vi "onSubscribe.vi"(6 "timeout (100ms)":i32=100, 8 "error in (no error)":errorcluster, 10 "SUBSCRIBE":refnum<class "SUBSCRIBE.lvclass">, 11 "MQTT_Base in":refnum<class "MQTT_Base.lvclass">) -> (0 "error out":errorcluster, 2 "SUBACK":refnum<class "SUBACK.lvclass">, 3 "MQTT_Base out":refnum<class "MQTT_Base.lvclass">)   [LabVIEW 2013, in "MQTT Base.lvlib" / "MQTT_Base.lvclass"]
uses:
  MQTT_Base.lvclass
  <vilib>/LabVIEW Open Source Project/MQTT Control Packets/Control Packets/SUBSCRIBE/SUBSCRIBE.lvclass
  <vilib>/LabVIEW Open Source Project/MQTT Control Packets/Control Packets/SUBACK/SUBACK.lvclass
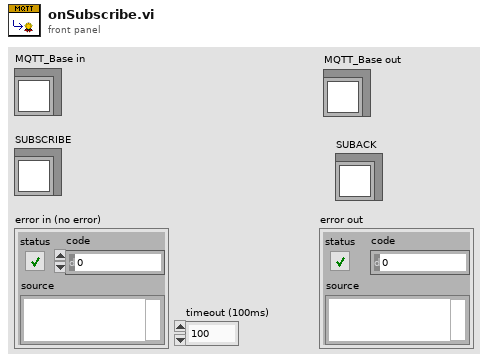
[diagram p1: front panel]
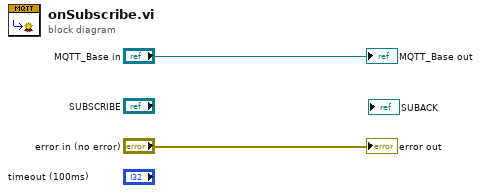
[diagram p0: block diagram]
diagram:
  "error out" <- "error in (no error)"
  "MQTT_Base out" <- "MQTT_Base in"
